vi "array sales ex 2.vi"() -> ()   [LabVIEW 2020]
panel:
  out "x*y":dbl[](array[numeric])
  out "subarray 2":string[](array[string])
  out "subarray":string[](array[string])
  out "array w/ subset deleted":string[][](array[string])
  out "sales data":string[][](array[string])
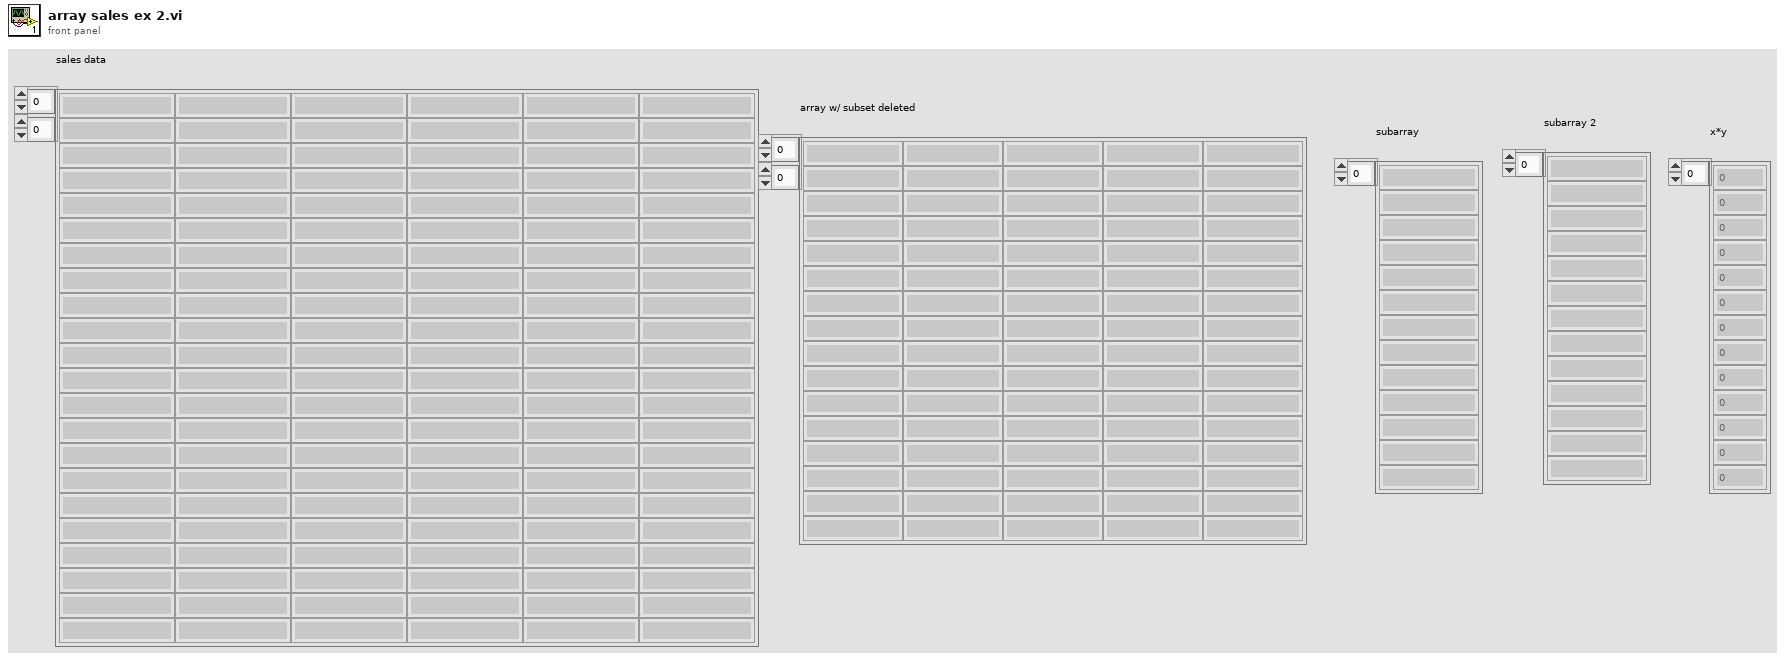
[diagram p1: front panel]
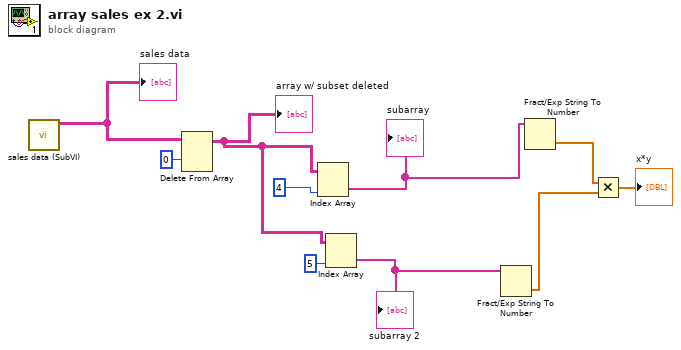
[diagram p0: block diagram]
diagram:
  n1 = call "sales data (SubVI).vi"() -> ("sales data"=w10:string[][])  [unwired: 11 in]
  "sales data" <- w10
  n2 = Delete From Array "Delete From Array"(array=w10, index (row)=0) -> (array with subset deleted=w8:string[][])  [unwired: 2 in, 1 out]
  "array w/ subset deleted" <- w8
  n3 = Index Array(array=w8, index (col)=4 ("index (row)")) -> (element=w5:string[])  [unwired: 1 in]
  "subarray" <- w5
  n4 = Index Array(array=w8, index (col)=5 ("disabled index (col)")) -> (element=w4:string[])  [unwired: 1 in]
  "subarray 2" <- w4
  n5 = Fract/Exp String To Number(string=w4) -> (number=w2:dbl[])  [unwired: 3 in, 1 out]
  n6 = Fract/Exp String To Number(string=w5) -> (number=w3:dbl[])  [unwired: 3 in, 1 out]
  n7 = Multiply(x=w3, y=w2) -> (x*y=→"x*y":dbl[])
